vi "Scannig-Probe-Microscope-Controller-2010-03-08-RFR-1a-version-for-MCL-drift-trial-fm-multiple-channels-nanoh50.vi"() -> ()   [LabVIEW 2012]
uses:
  <vilib>/rvi/eio/common/nirviEmuTemplateMethod_errors.vi
  <vilib>/rvi/Emulation/niFpgaSctlEmulationGetInTimedLoop.vi
  <vilib>/rvi/Emulation/niFpgaSctlEmulationGlobalWrite.vi
  <vilib>/rvi/interface/RandomDataEmulation/nirviRandomDataFPGAFIFO.vi
  <vilib>/rvi/interface/RandomDataEmulation/niFpgaRandomDataHandleErrors.vi
  <vilib>/eio/EIONode/EIONode.xnode
  <vilib>/rvi/Analysis/measure/butterworth/XNode/niFpgaButterworthFilter.xnode
  <vilib>/rvi/DataTransferAndStorage/Container/XNode/niFpgaContainer.xnode
  <vilib>/rvi/interface/RandomDataEmulation/nirviRandomDataFpgaReadWriteTemplate.vi
panel:
  in  "Direction":bool
  in  "Enable":bool
  out "Dir":bool
  out "En":bool
  in  "Change Dir / Enable":bool
  in  "Stepper Motor Stop":bool
  in  "Step Motor Cycle (usec)":u32 caption="Stepper Motor Cycle"
  out "Step":bool
  in  "Manual-fixed-steps":i32
  in  "Continuous/Fixed":bool
  in  "Stepper Motor":bool
  in  "Timeout":i32=-1
  in  "acquisition rate calibration":u32 caption="Count(uSec)"
  in  "Manual control Output Calibration":i16
  in  "Wait before\ncalibration":u32 caption="Count(uSec)"
  in  "Size-calibration":i32
  in  "Calibration-period":u32 caption="Count(uSec)"
  in  "Initial Position\n Calibration":i32
  in  "AO1":i16
  in  "Start calibration":bool
  out "AI4":i16
  out "AI2":i16
  out "AI6":i16
  out "AI5":i16
  in  "P scale":i8=-1
  in  "offset retraction drift":i16
  in  "time before averaging drift":u32 caption="Count(uSec)"
  in  "Setpoint Control":bool
  in  "Internal Setpoint Internal Control":i16
  in  "Internal Setpoint External Control":i16=357
  in  "Stop Feedback Control":bool
  in  "shift integrator control":i32
  in  "shift integrator":i32
  out "offset out":i16
  in  "drift temporal control":u32
  in  "offset FM":u16
  in  "drift averager":u16
  out "TF-drift":i16
  out "Counter Data":i8 min=-1 step=1
  in  "drift Waiting (uSec)":u16
  out "End of image":bool
  in  "Pixels in one image":i32
  in  "Scanning Y indicator":bool
  in  "Stop Feedback":bool
  in  "Steps per Feedback Region":i32=665
  in  "Y Number of Lines":u32=10
  in  "PID gains (x 2^8)":T1={"proportional gain (Kc)"=1, "integral gain (Kc*Ts/Ti)"=0, "derivative gain (Kc*Td/Ts)"=0}
  out "Command Out":i16=-4104
  in  "provisional limit":i8=102
  out "accumulator limit":i8=-1
  in  "shift-divisions (always >=2)":i8=100
  out "limit indicator":u8
  in  "counter":i8 min=-1 step=1
  in  "Internal Setpoint":i16=357
  in  "I scale":i8=-1
  in  "Count(uSec)":u8=232
  in  "Timeout FIFO":i32=-1
  out "Y line":i32
  out "iterations x":i32
  out "X Output Value":i16=3
  in  "Forth/Back Y axis":bool
  out "Inidicator \nforth/back  Y axis":i8=1
  in  "Time per step/\nX axis sub pixel (uSec)":u16=31 caption="Count(uSec)"
  in  "Time per image pixel/\nX axis pixel (uSec)":u16=1984 caption="Count(uSec)"
  in  "Time per step/\nY axis sub pixel (uSec)":u32=7936 caption="Count(uSec)"
  out "Y Output Value":i16=32702
  out "End of scan line?":bool
  in  "Forth/Back X axis":bool
  in  "Image Total Pixels":u32=65536
  out "Indicator \nforth/back X axis":i8=1
  in  "Y axis pixels":u16=255
  in  "Y steps per pixel":u16=64
  in  "X steps per pixel":u16=64
  in  "y initial":i16
  in  "x initial":i16
  in  "X axis pixels":u16=255
  in  "Scanning On/Off":bool
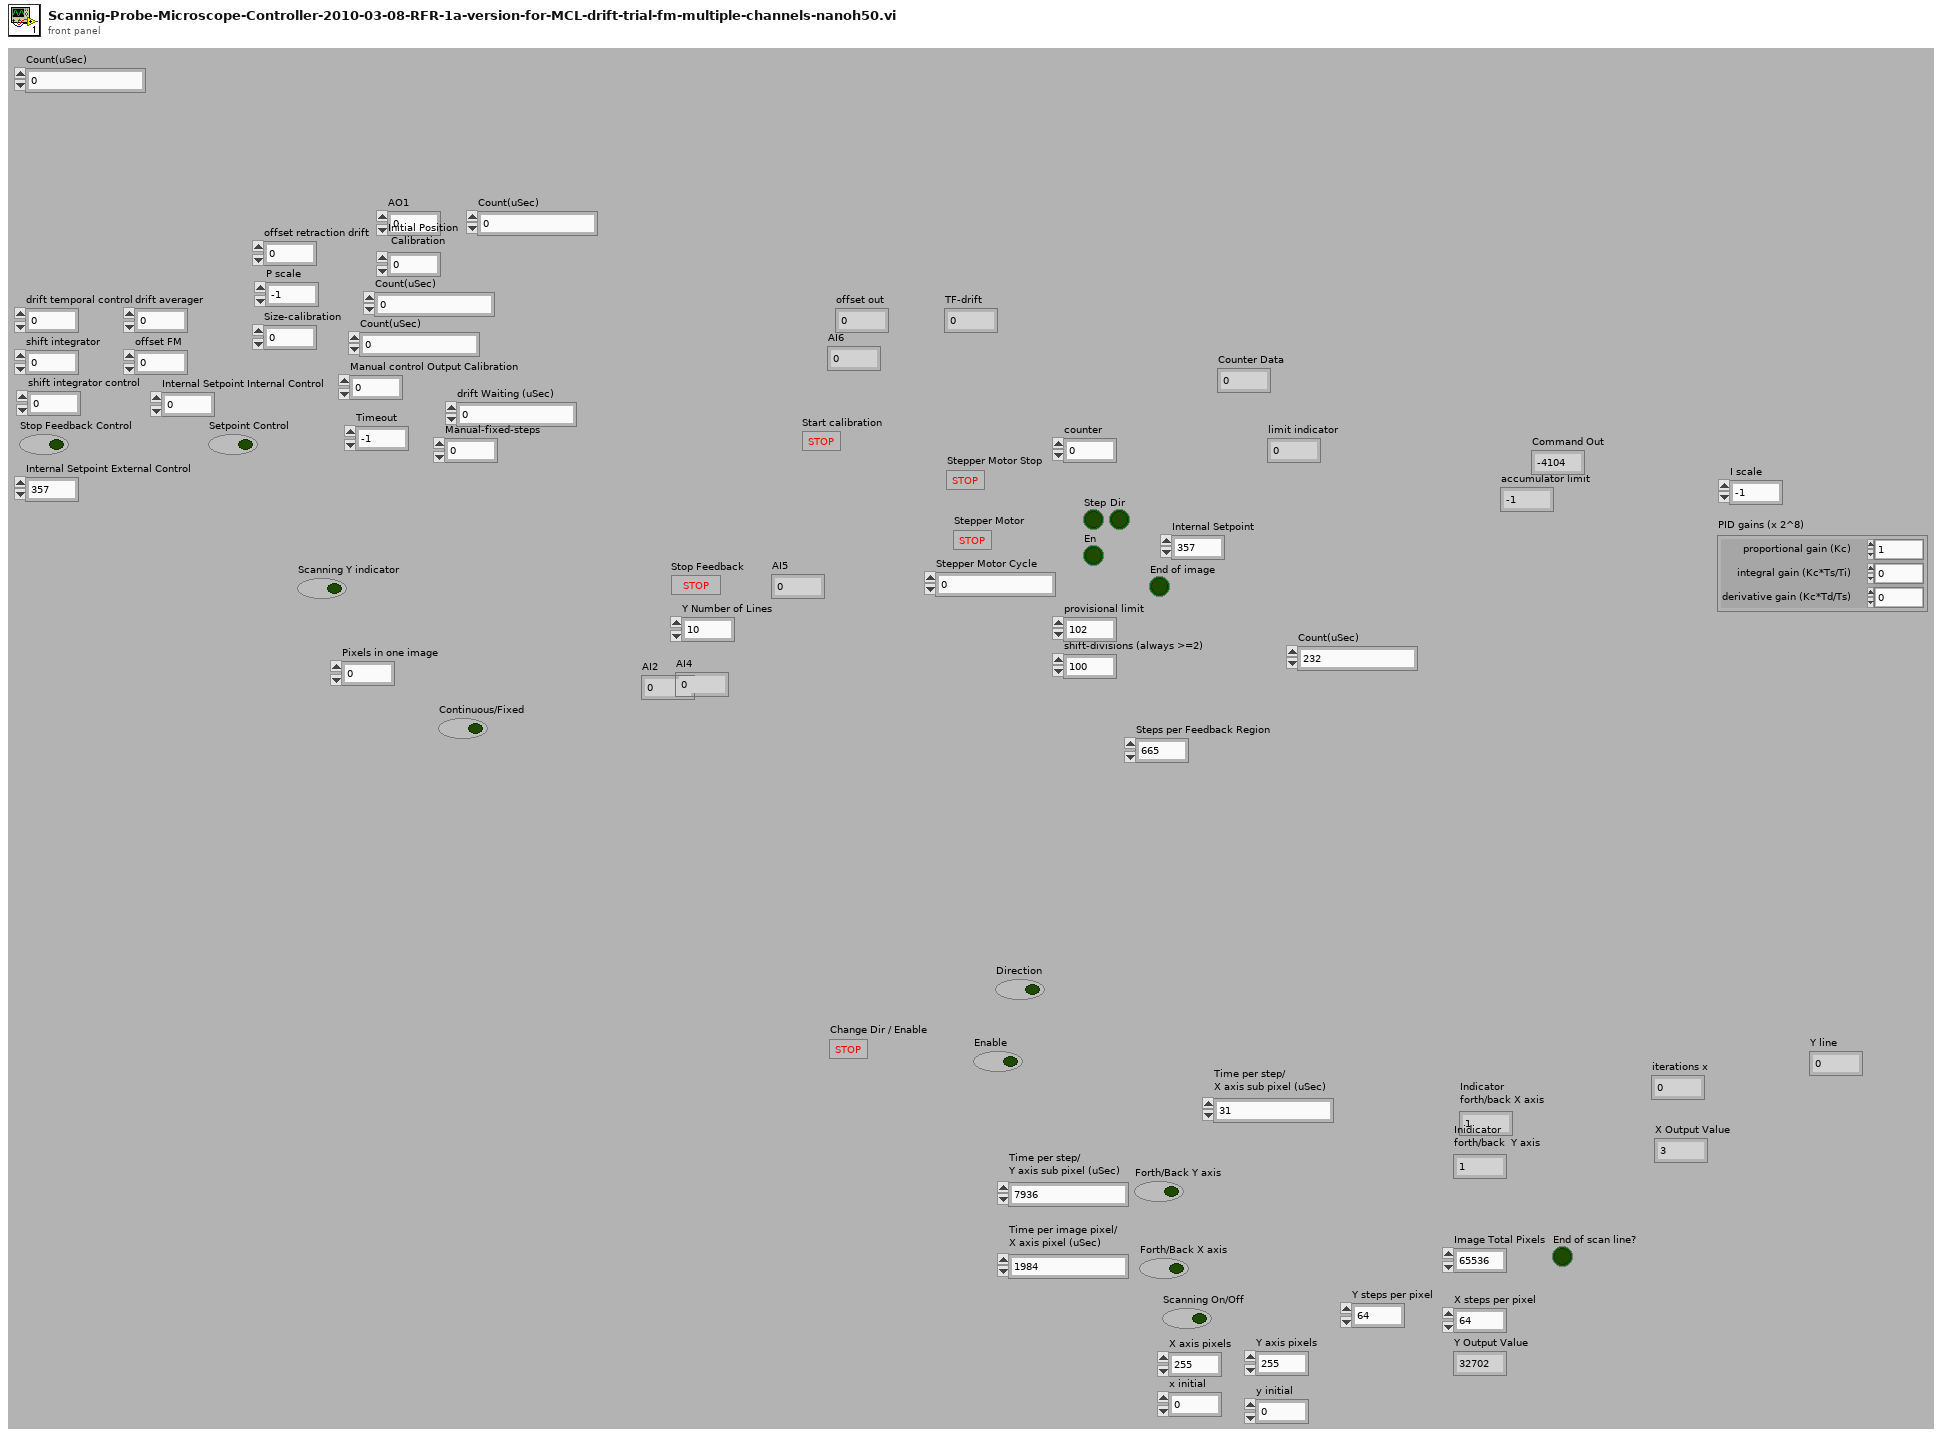
[diagram p1: front panel]
types:
  T1 = cluster{"proportional gain (Kc)":i16, "integral gain (Kc*Ts/Ti)":i16, "derivative gain (Kc*Td/Ts)":i16}
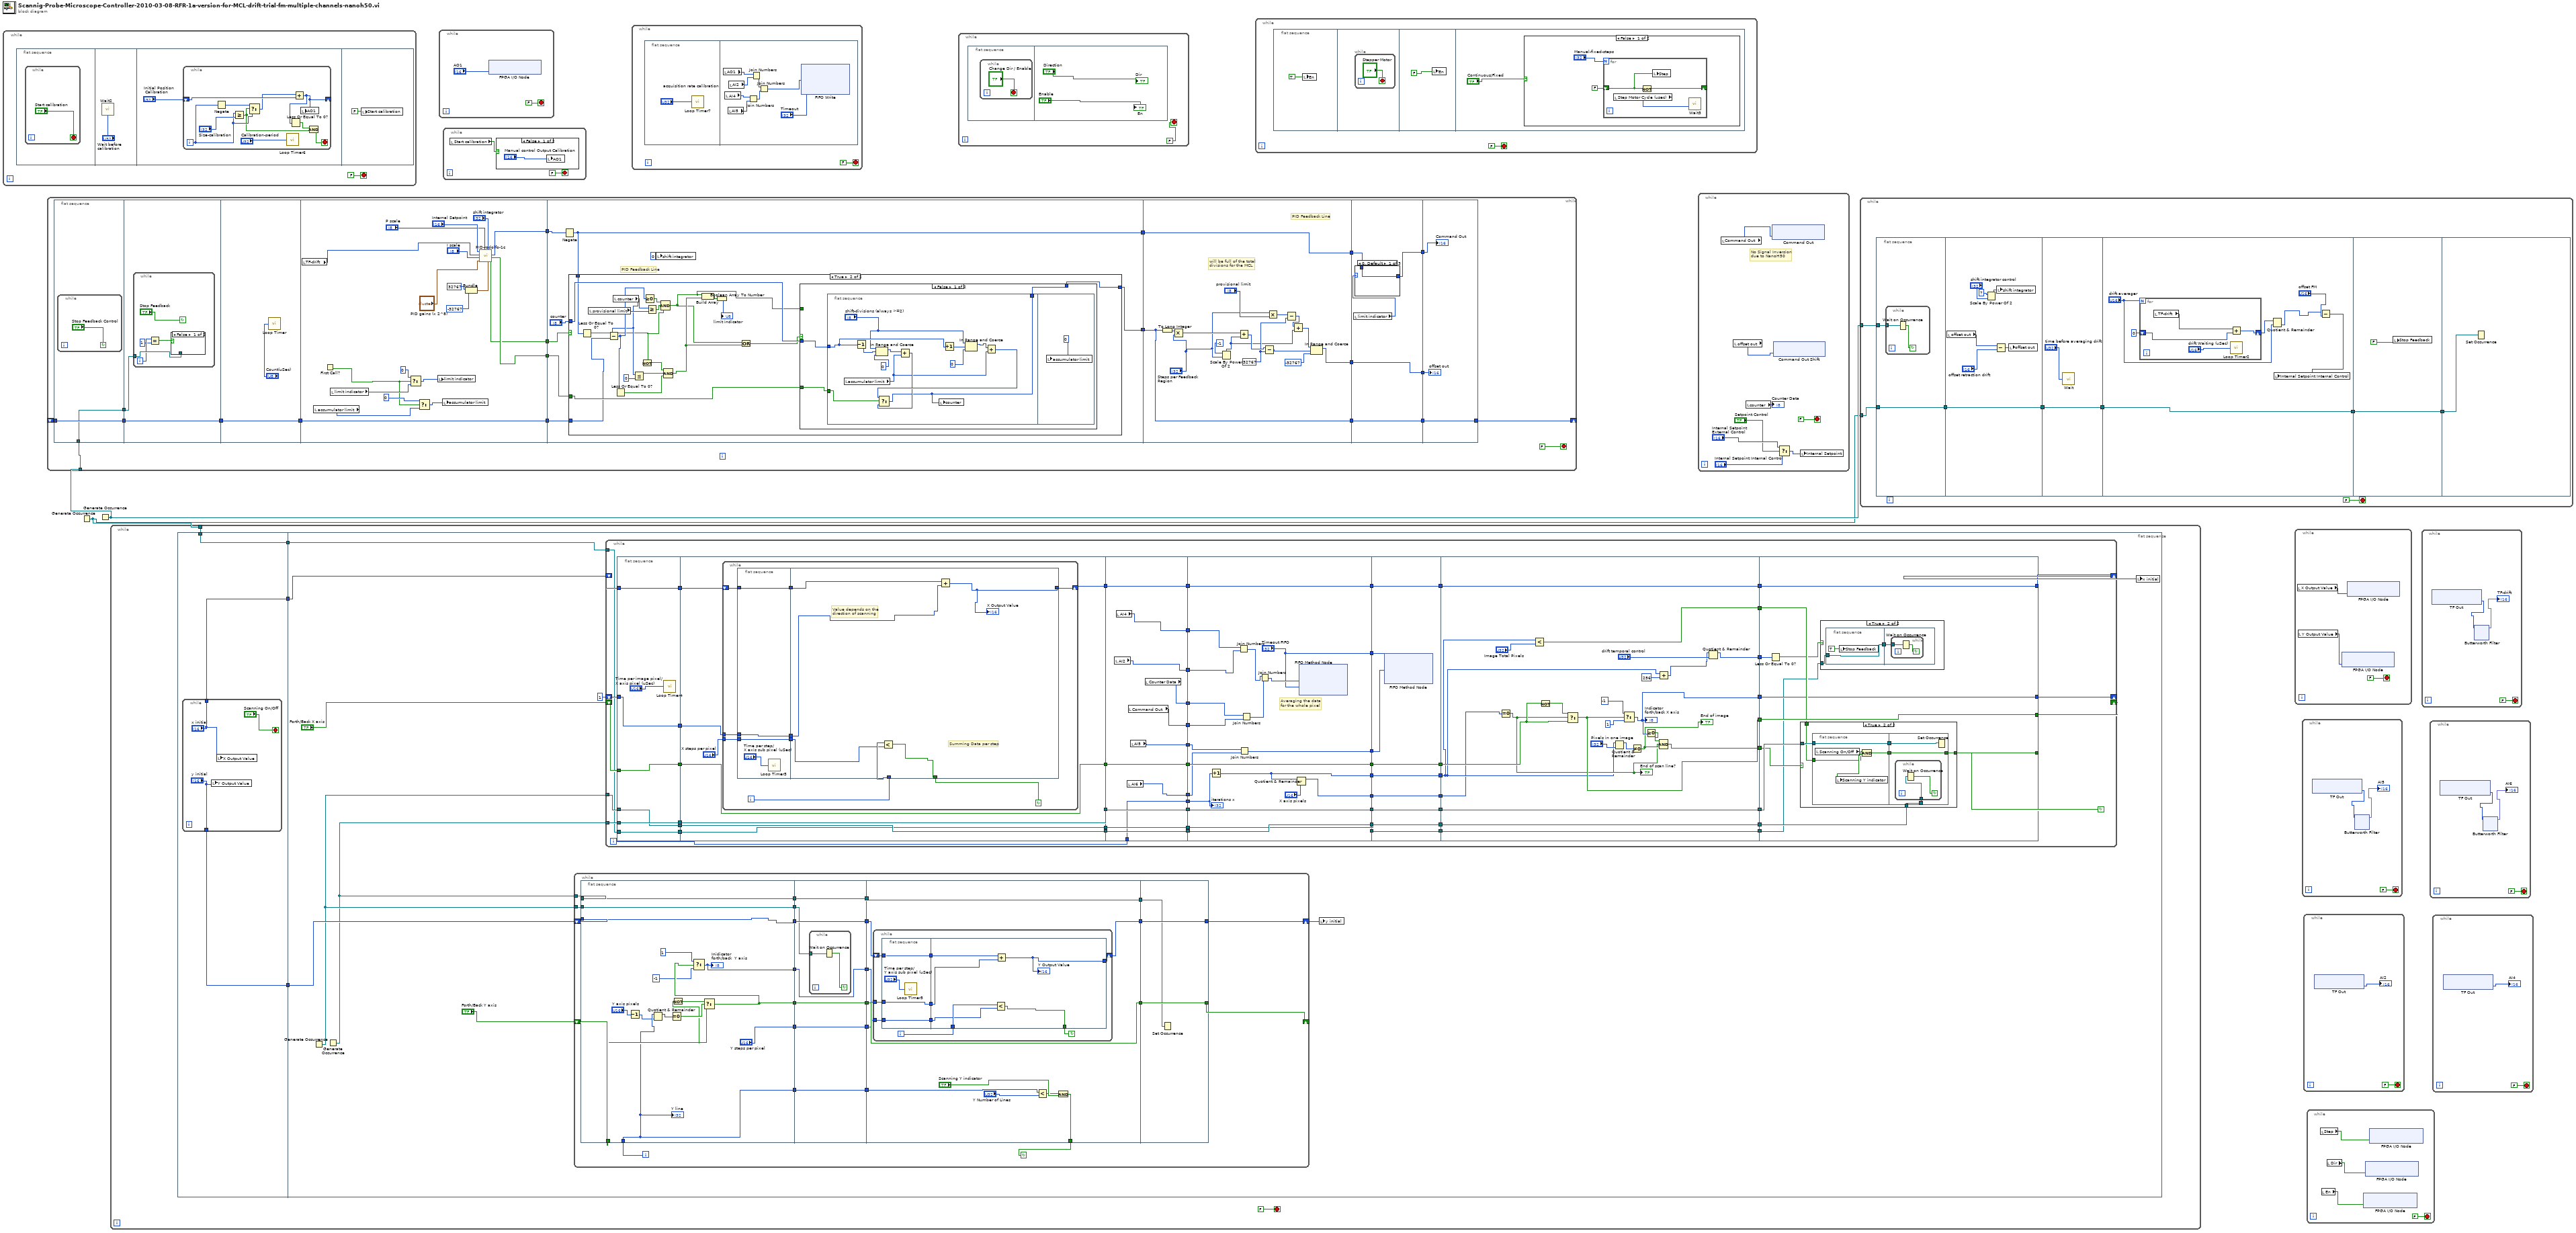
[diagram p0: block diagram]
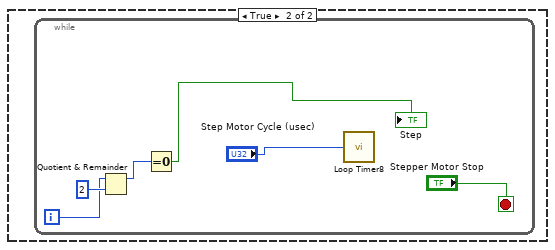
[diagram p2: hidden frame]
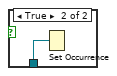
[diagram p4: hidden frame]
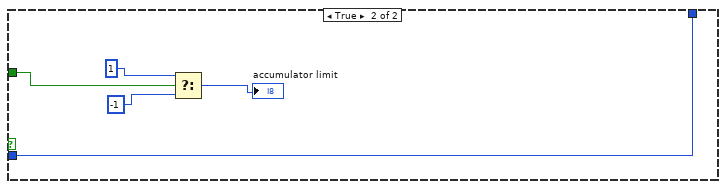
[diagram p6: hidden frame]
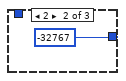
[diagram p7: hidden frame]
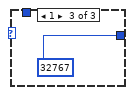
[diagram p8: hidden frame]
diagram:
  n1 = while {
    stop <- FALSE stop-if-true
    n2 = flat-sequence {
      frame #0 {
        n3 = while {
          stop <- "Start calibration" stop-if-true
        }
      }
      frame #1 {
        n4 = call "Wait2"("Count(uSec)"="Wait before\ncalibration") -> ()  [unwired: 1 out]
      }
      frame #2 {
        n5 = while {
          shift-right: [w10] -> _
          shift-left: "Initial Position\n Calibration" -> [w16]
          i -> [w11]
          stop <- w7 stop-if-true
          n6 = Negate(x=w11) -> (-x=w14:i32)
          n7 = Greater Or Equal?(x=w11, y="Size-calibration") -> (x >= y?=w8:bool)
          n8 = Select(t=w14, s=w8, f=w11) -> (s? t:f=w12:i32)
          n9 = call "Loop Timer6"("Count(uSec)"="Calibration-period") -> ()  [unwired: 1 out]
          n10 = Add(x=w12, y=w16) -> (x+y=w10:i32)
          n11 = Less Or Equal To 0?(x=w10) -> (x <= 0?=w9:bool)
          n12 = local write "AO1"(w10) -> ()
          n13 = Compound Arithmetic op=AND(w9, w8) -> (w7:bool)
        }
      }
      frame #3 {
        n14 = local write "Start calibration"(FALSE ("Start calibration")) -> ()
      }
    }
  }
  n15 = Generate Occurrence() -> (w1:refnum<k4>)
  n16 = Generate Occurrence() -> (w2:refnum<k4>)
  n17 = while {
    shift-right: [w28] -> _
    shift-left: _ -> [w27]
    tunnel: w2 -> [w19]
    stop <- FALSE stop-if-true
    n18 = flat-sequence {
      tunnel: w27 -> [w39]
      tunnel: [w39] -> w21
      tunnel: w19 -> [w38]
      tunnel: [w38] -> w18
      tunnel: w21 -> [w42]
      tunnel: [w42] -> w20
      tunnel: w18 -> [w41]
      tunnel: [w49] -> w26
      tunnel: w20 -> [w49]
      tunnel: [w67] -> w25
      tunnel: [w66] -> w24
      tunnel: [w65] -> w23
      tunnel: w26 -> [w62]
      tunnel: [w62] -> w22
      tunnel: [w78] -> w31
      tunnel: w25 -> [w77]
      tunnel: [w73] -> w32
      tunnel: w24 -> [w75]
      tunnel: w23 -> [w74]
      tunnel: w22 -> [w72]
      tunnel: w32 -> [w135]
      tunnel: [w135] -> w34
      tunnel: w31 -> [w132]
      tunnel: [w133] -> w33
      tunnel: [w132] -> w30
      tunnel: [w139] -> w36
      tunnel: w34 -> [w141]
      tunnel: [w142] -> w35
      tunnel: w33 -> [w139]
      tunnel: w30 -> [w138]
      tunnel: [w138] -> w29
      tunnel: w36 -> [w146]
      tunnel: w35 -> [w148]
      tunnel: w29 -> [w147]
      tunnel: [w147] -> w28
      frame #0 {
        n19 = while {
          stop <- "Stop Feedback Control" continue-if-true
        }
      }
      frame #1 {
        n20 = while {
          tunnel: w41 -> [w47]
          i -> [w45]
          stop <- "Stop Feedback" continue-if-true
          n21 = Equal?(x=w45, y=u8 1) -> (x = y?=w43:bool)
          n22 = case shown="False" w43 {
            tunnel: w47 -> [_ w48]
            frame False {
            }
            frame True {
              n23 = Set Occurrence(w48) -> ()
            }
          }
        }
      }
      frame #2 {
        n24 = call "Loop Timer"("Count(uSec)"="Count(uSec)") -> ()  [unwired: 1 out]
      }
      frame #3 {
        n25 = local read "TF-drift"() -> (w52:i16)
        n26 = local read "accumulator limit"() -> (w55:i8)
        n27 = First Call?() -> (First Call?: T/F=w53:bool)
        n28 = local read "limit indicator"() -> (w58:u8)
        n29 = Select(t=u8 0, s=w53, f=w58) -> (s? t:f=w59:u8)
        n30 = Select(t=i8 0, s=w53, f=w55) -> (s? t:f=w57:i8)
        n31 = local write "limit indicator"(w59) -> ()
        n32 = local write "accumulator limit"(w57) -> ()
        n33 = Bundle(i16 32767, i16 -32767) -> (w68:cluster{i16, i16})  [unwired: 1 in]
        n34 = call "PID-rodolfo-1c.vi"("output range"=w68, "shift integrator"="shift integrator", "P scale"="P scale", "PID gains (x 2^8)"="PID gains (x 2^8)", "I scale"="I scale", "process variable"=w52, "setpoint"="Internal Setpoint") -> ("yes/no"=w65:bool, "upper/lower"=w66:bool, "output"=w67:i16)  [unwired: 2 in]
      }
      frame #4 {
        # "PID Feedback Line"
        n35 = Negate(x=w77) -> (-x=w73:i16)
        n36 = case shown="True" w74 {
          tunnel: "counter" -> [w79 w99]
          tunnel: [w79 w98] -> w78
          tunnel: w75 -> [_ w82]
          tunnel: w73 -> [_ w87]
          tunnel: w72 -> [_ w80]
          frame False {
          }
          frame True {
            n37 = Less Or Equal To 0?(x=w87) -> (x <= 0?=w88:bool)
            n38 = local read "provisional limit"() -> (w95:i8)
            n39 = local read "counter"() -> (w90:i8)
            n40 = Subtract(x=w90, y=w80) -> (x-y=w91:i8)
            n41 = Less Or Equal To 0?(x=w91) -> (x <= 0?=w92:bool)
            n42 = Less Or Equal?(x=w90, y=u8 0) -> (x <= y?=w93:bool)
            n43 = Not(x=w88) -> (.not. x?=w89:bool)
            n44 = Greater Or Equal To 0?(x=w91) -> (x >= 0?=w97:bool)
            n45 = Greater Or Equal?(x=w90, y=w95) -> (x >= y?=w96:bool)
            n46 = Compound Arithmetic op=AND(w97, w96, w88) -> (w81:bool)
            n47 = Compound Arithmetic op=AND(w89, w93, w92) -> (w84:bool)
            n48 = Build Array(w81, w84) -> (w86:bool[])
            n49 = Boolean Array To Number(Boolean array=w86) -> (number=→"limit indicator":u8)
            n50 = Or(x=w81, y=w84) -> (x .or. y?=w83:bool)
            n51 = case shown="False" w83 {
              tunnel: w99 -> [w102 w121]
              tunnel: [w101 w121] -> w98
              tunnel: w82 -> [w100 _]
              tunnel: w81 -> [_ w117]
              frame False {
                n52 = flat-sequence {
                  tunnel: w102 -> [w108]
                  tunnel: [w105] -> w101
                  tunnel: w100 -> [w109]
                  frame #0 {
                    n53 = local read "accumulator limit"() -> (w104:i8)
                    n54 = Decrement(x=w108) -> (x-1=w112:i8)
                    n55 = In Range and Coerce(upper limit="shift-divisions (always >=2)", x=w112, lower limit=i8 0) -> (coerced(x)=w110:i8)  [unwired: 1 out]
                    n56 = Add(x=w110, y=w104) -> (x+y=w106:i8)
                    n57 = Increment(x=w108) -> (x+1=w113:i8)
                    n58 = In Range and Coerce(upper limit="shift-divisions (always >=2)", x=w113, lower limit=i8 0 ("y")) -> (coerced(x)=w115:i8)  [unwired: 1 out]
                    n59 = Add(x=w115, y=w104) -> (x+y=w107:i8)
                    n60 = Select(t=w107, s=w109, f=w106) -> (s? t:f=w105:i8)
                    n61 = local write "counter"(w105) -> ()
                  }
                  frame #1 {
                    n62 = local write "accumulator limit"(i8 0 ("accumulator limit")) -> ()
                  }
                }
              }
              frame True {
                n63 = Select(t=i8 1, s=w117, f=i8 -1) -> (s? t:f=→"accumulator limit":i8)
              }
            }
          }
        }
        n64 = local write "shift integrator"(0 ("new integrator")) -> ()
      }
      frame #5 {
        w125 = 32767 ("y")
        # "PID Feedback Line"
        # "will be full of the total\ndivisions for the MCL"
        n65 = To Long Integer(number=w132) -> (32bit integer=w131:i32)
        n66 = Multiply(x=w131, y="Steps per Feedback Region") -> (x*y=w136:i32)
        n67 = Scale By Power Of 2(n=i8 -1, x="Steps per Feedback Region") -> (x*2^n=w124:i32)
        n68 = Add(x=w136, y=w124) -> (x+y=w128:i32)
        n69 = Subtract(x=w128, y=w125) -> (x-y=w127:i32)
        n70 = Multiply(x="Steps per Feedback Region", y="provisional limit") -> (x*y=w126:i32)
        n71 = Subtract(x=w126, y=w125) -> (x-y=w123:i32)
        n72 = Add(x=w123, y=w124) -> (x+y=w122:i32)
        n73 = In Range and Coerce(upper limit=w122, x=w127, lower limit=-32767) -> (coerced(x)=w133:i32)  [unwired: 1 out]
      }
      frame #6 {
        n74 = local read "limit indicator"() -> (w140:u8)
        n75 = case shown="0, Default" w140 {
          tunnel: w141 -> [w143 _ _]
          tunnel: [w143 i16 -32767 i16 32767] -> w142
          frame 0, Default {
          }
          frame 2 {
          }
          frame 1 {
          }
        }
      }
      frame #7 {
        "Command Out" <- w148
        "offset out" <- w146
      }
    }
  }
  n76 = while {
    tunnel: w1 -> [w149]
    stop <- FALSE stop-if-true
    n77 = flat-sequence {
      tunnel: [w155] -> w152
      tunnel: [w156] -> w151
      tunnel: [w154] -> w150
      tunnel: w149 -> [w154]
      tunnel: w152 -> [w165]
      tunnel: w151 -> [w164]
      tunnel: w150 -> [w160]
      frame #0 {
        n78 = while {
          tunnel: ["y initial"] -> w156
          tunnel: ["x initial"] -> w155
          stop <- "Scanning On/Off" stop-if-true
          n79 = local write "Y Output Value"("y initial") -> ()
          n80 = local write "X Output Value"("x initial") -> ()
        }
      }
      frame #1 {
        n81 = Generate Occurrence() -> (w163:refnum<k4>)
        n82 = Generate Occurrence() -> (w162:refnum<k4>)
        n83 = while {
          shift-right: [w193] -> _
          shift-left: "Forth/Back Y axis" -> [w192]
          shift-right: [w190] -> w166
          shift-left: w164 -> [w191]
          tunnel: w163 -> [w189]
          tunnel: w162 -> [w185]
          i -> [w173]
          stop <- w172 continue-if-true
          n84 = flat-sequence {
            tunnel: w192 -> [w206]
            tunnel: [w204] -> w184
            tunnel: [w201] -> w182
            tunnel: [w200] -> w180
            tunnel: [w199] -> w178
            tunnel: ["Y steps per pixel"] -> w176
            tunnel: [w197] -> w174
            tunnel: w173 -> [w196]
            tunnel: w191 -> [w201]
            tunnel: w185 -> [w199]
            tunnel: w189 -> [w197]
            tunnel: [w196] -> w170
            tunnel: w184 -> [w215]
            tunnel: [w215] -> w183
            tunnel: w182 -> [w214]
            tunnel: [w214] -> w181
            tunnel: w180 -> [w213]
            tunnel: [w213] -> w179
            tunnel: w178 -> [w212]
            tunnel: [w212] -> w177
            tunnel: w176 -> [w211]
            tunnel: [w211] -> w175
            tunnel: w174 -> [w210]
            tunnel: [w209] -> w171
            tunnel: w170 -> [w209]
            tunnel: w183 -> [w228]
            tunnel: w181 -> [w227]
            tunnel: w179 -> [w225]
            tunnel: [w228] -> w188
            tunnel: [w226] -> w187
            tunnel: [w224] -> w186
            tunnel: w177 -> [w224]
            tunnel: w175 -> [w223]
            tunnel: [w219] -> w172
            tunnel: w171 -> [w218]
            tunnel: [w249] -> w190
            tunnel: [w250] -> w193
            tunnel: w188 -> [w250]
            tunnel: w187 -> [w249]
            tunnel: w186 -> [w248]
            frame #0 {
              n85 = Decrement(x="Y axis pixels") -> (x-1=w194:u16)
              n86 = Quotient & Remainder(x=w196, y=w194) -> (x-y*floor(x/y)=w208:i32)  [unwired: 1 out]
              n87 = Equal To 0?(x=w208) -> (x = 0?=w207:bool)
              n88 = Not(x=w206) -> (.not. x?=w205:bool)
              n89 = Select(t=w205, s=w207, f=w206) -> (s? t:f=w204:bool)
              n90 = Select(t=i8 1, s=w204, f=i8 -1 ("Inidicator \nforth/back  Y axis")) -> (s? t:f=w200:i8)
              "Inidicator \nforth/back  Y axis" <- w200
              "Y line" <- w196
            }
            frame #1 {
              n91 = while {
                tunnel: w210 -> [w216]
                stop <- w217 continue-if-true
                n92 = Wait on Occurrence(2:w216) -> (0:w217:bool)  [unwired: 2 in]
              }
            }
            frame #2 {
              n93 = while {
                shift-right: [w234] -> w226
                shift-left: w227 -> [w235]
                tunnel: w225 -> [w231]
                tunnel: w223 -> [w229]
                i -> [w236]
                stop <- w237 continue-if-true
                n94 = flat-sequence {
                  tunnel: w235 -> [w241]
                  tunnel: [w241] -> w233
                  tunnel: [w239] -> w232
                  tunnel: w231 -> [w239]
                  tunnel: [w238] -> w230
                  tunnel: w229 -> [w238]
                  tunnel: [w243] -> w237
                  tunnel: w236 -> [w247]
                  tunnel: [w245] -> w234
                  tunnel: w233 -> [w246]
                  tunnel: w232 -> [w244]
                  tunnel: w230 -> [w242]
                  frame #0 {
                    n95 = call "Loop Timer5"("Count(uSec)"="Time per step/\nY axis sub pixel (uSec)") -> ()  [unwired: 1 out]
                  }
                  frame #1 {
                    n96 = Less?(x=w247, y=w242) -> (x < y?=w243:bool)
                    n97 = Add(x=w246, y=w244) -> (x+y=w245:i16)
                    "Y Output Value" <- w245
                  }
                }
              }
              n98 = Less?(x=w218, y="Y Number of Lines") -> (x < y?=w220:bool)
              n99 = Compound Arithmetic op=AND(w220, "Scanning Y indicator") -> (w219:bool)
            }
            frame #3 {
              n100 = Set Occurrence(w248) -> ()
            }
          }
        }
        n101 = while {
          shift-right: [w307] -> w167
          shift-left: w165 -> [w309]
          shift-right: [w294] -> _
          shift-left: "Forth/Back X axis" -> [w308]
          tunnel: w163 -> [w306]
          tunnel: w162 -> [w305]
          shift-right: [w296] -> _
          shift-left: i8 1 ("Indicator \nforth/back") -> [w295]
          tunnel: w160 -> [w275]
          i -> [w267]
          stop <- w304 continue-if-true
          n102 = flat-sequence {
            tunnel: w308 -> [w315]
            tunnel: w309 -> [w316]
            tunnel: [w316] -> w293
            tunnel: [w315] -> w292
            tunnel: w306 -> [w313]
            tunnel: [w313] -> w291
            tunnel: [w312] -> w290
            tunnel: w305 -> [w312]
            tunnel: [w311] -> w289
            tunnel: w295 -> [w311]
            tunnel: w275 -> [w310]
            tunnel: [w310] -> w271
            tunnel: w293 -> [w322]
            tunnel: [w324] -> w288
            tunnel: [w321] -> w282
            tunnel: w290 -> [w321]
            tunnel: [w320] -> w280
            tunnel: w291 -> [w320]
            tunnel: [w319] -> w278
            tunnel: w292 -> [w319]
            tunnel: w289 -> [w323]
            tunnel: [w317] -> w272
            tunnel: w271 -> [w317]
            tunnel: w288 -> [w355]
            tunnel: [w355] -> w287
            tunnel: [w344] -> w286
            tunnel: [w345] -> w285
            tunnel: [w350] -> w284
            tunnel: [w351] -> w283
            tunnel: w282 -> [w354]
            tunnel: [w354] -> w281
            tunnel: w280 -> [w353]
            tunnel: [w353] -> w279
            tunnel: w278 -> [w352]
            tunnel: [w352] -> w277
            tunnel: [w349] -> w273
            tunnel: w272 -> [w349]
            tunnel: [w346] -> w270
            tunnel: [w347] -> w269
            tunnel: [w348] -> w268
            tunnel: w267 -> [w348]
            tunnel: w287 -> [w375]
            tunnel: w286 -> [w367]
            tunnel: w285 -> [w366]
            tunnel: w284 -> [w371]
            tunnel: w283 -> [w365]
            tunnel: [w375] -> w266
            tunnel: [w370] -> w264
            tunnel: w281 -> [w370]
            tunnel: [w369] -> w262
            tunnel: w279 -> [w369]
            tunnel: [w368] -> w260
            tunnel: w277 -> [w368]
            tunnel: [w364] -> w258
            tunnel: w273 -> [w364]
            tunnel: w270 -> [w363]
            tunnel: w269 -> [w362]
            tunnel: w268 -> [w361]
            tunnel: [w359] -> w256
            tunnel: [w358] -> w254
            tunnel: ["Timeout FIFO"] -> w252
            tunnel: [w356] -> w251
            tunnel: w266 -> [w384]
            tunnel: [w384] -> w265
            tunnel: w264 -> [w383]
            tunnel: [w383] -> w263
            tunnel: w262 -> [w382]
            tunnel: [w382] -> w261
            tunnel: w260 -> [w381]
            tunnel: [w381] -> w259
            tunnel: w258 -> [w380]
            tunnel: [w380] -> w257
            tunnel: w256 -> [w379]
            tunnel: [w379] -> w255
            tunnel: w254 -> [w378]
            tunnel: [w378] -> w253
            tunnel: w252 -> [w377]
            tunnel: w251 -> [w376]
            tunnel: [w400] -> w303
            tunnel: w265 -> [w408]
            tunnel: [w408] -> w302
            tunnel: w263 -> [w407]
            tunnel: [w407] -> w301
            tunnel: w261 -> [w406]
            tunnel: [w406] -> w300
            tunnel: [w401] -> w299
            tunnel: w259 -> [w399]
            tunnel: [w398] -> w298
            tunnel: [w397] -> w297
            tunnel: [w390] -> w276
            tunnel: [w387] -> w274
            tunnel: w257 -> [w387]
            tunnel: w255 -> [w386]
            tunnel: w253 -> [w385]
            tunnel: [w418] -> w307
            tunnel: [w419] -> w294
            tunnel: w303 -> [w419]
            tunnel: w302 -> [w418]
            tunnel: w301 -> [w417]
            tunnel: w300 -> [w416]
            tunnel: w299 -> [w415]
            tunnel: [w414] -> w304
            tunnel: w298 -> [w413]
            tunnel: [w412] -> w296
            tunnel: w297 -> [w412]
            tunnel: w276 -> [w411]
            tunnel: w274 -> [w409]
            frame #0 {
              n103 = call "Loop Timer4"("Count(uSec)"="Time per image pixel/\nX axis pixel (uSec)") -> ()  [unwired: 1 out]
            }
            frame #1 {
              n104 = while {
                shift-right: [w330] -> w324
                shift-left: w322 -> [w331]
                tunnel: w323 -> [w327]
                tunnel: "X steps per pixel" -> [w325]
                i -> [w332]
                stop <- w333 continue-if-true
                n105 = flat-sequence {
                  tunnel: w331 -> [w337]
                  tunnel: [w337] -> w329
                  tunnel: [w335] -> w328
                  tunnel: w327 -> [w335]
                  tunnel: [w334] -> w326
                  tunnel: w325 -> [w334]
                  tunnel: [w339] -> w333
                  tunnel: w332 -> [w343]
                  tunnel: [w341] -> w330
                  tunnel: w329 -> [w342]
                  tunnel: w328 -> [w340]
                  tunnel: w326 -> [w338]
                  frame #0 {
                    n106 = call "Loop Timer3"("Count(uSec)"="Time per step/\nX axis sub pixel (uSec)") -> ()  [unwired: 1 out]
                  }
                  frame #1 {
                    # "Summing Data per step"
                    # "Value depends on the\ndirection of scanning"
                    n107 = Less?(x=w343, y=w338) -> (x < y?=w339:bool)
                    n108 = Add(x=w342, y=w340) -> (x+y=w341:i16)
                    "X Output Value" <- w341
                  }
                }
              }
            }
            frame #2 {
              n109 = local read "AI2"() -> (w345:i16)
              n110 = local read "AI4"() -> (w344:i16)
              n111 = local read "AI6"() -> (w347:i16)
              n112 = local read "Command Out"() -> (w351:i16)
              n113 = local read "AI5"() -> (w346:i16)
              n114 = local read "Counter Data"() -> (w350:i8)
            }
            frame #3 {
              # "Averaging the data \nfor the whole pixel"
              n115 = Increment(x=w361) -> (x+1=w359:i32)
              n116 = Join Numbers(hi=w367, lo=w366) -> ((hi.lo)=w372:u32)
              n117 = Join Numbers(hi=w363, lo=w362) -> ((hi.lo)=w356:u32)
              n118 = Join Numbers(hi=w371, lo=w365) -> ((hi.lo)=w373:u32)
              n119 = Join Numbers(hi=w372, lo=w373) -> ((hi.lo)=w374:u64)
              n120 = Quotient & Remainder(x=w359, y="X axis pixels") -> (x-y*floor(x/y)=w358:i32)  [unwired: 1 out]
              n121 = xnode "FIFO Method Node"("Element"=w374, "Timeout"="Timeout FIFO") -> ()  [unwired: 1 in, 2 out]
              "iterations x" <- w361
            }
            frame #4 {
              n122 = xnode ("FIFO Method Node")("Element"=w376, "Timeout"=w377) -> ()  [unwired: 1 in, 2 out]
            }
            frame #5 {
              n123 = Equal To 0?(x=w385) -> (x = 0?=w393:bool)
              "End of scan line?" <- w393
              n124 = Less?(x=w386, y="Image Total Pixels") -> (x < y?=w401:bool)
              n125 = Not(x=w399) -> (.not. x?=w405:bool)
              n126 = Select(t=w405, s=w393, f=w399) -> (s? t:f=w400:bool)
              n127 = Quotient & Remainder(x=w386, y="Pixels in one image") -> (x-y*floor(x/y)=w394:i32)  [unwired: 1 out]
              n128 = Select(t=i8 -1 ("Indicator \nforth/back"), s=w400, f=i8 1 ("Indicator \nforth/back")) -> (s? t:f=w397:i8)
              "Indicator \nforth/back X axis" <- w397
              n129 = Not Equal To 0?(x=w394) -> (x != 0?=w396:bool)
              "End of image" <- w396
              n130 = Greater Or Equal To 0?(x=w397) -> (x >= 0?=w392:bool)
              n131 = Add(x=w386, y=u16 256) -> (x+y=w388:i32)
              n132 = Compound Arithmetic op=AND(w392, w393, w396) -> (w398:bool)
              n133 = Quotient & Remainder(x=w388, y="drift temporal control") -> (x-y*floor(x/y)=w390:u32)  [unwired: 1 out]
            }
            frame #6 {
              n134 = Less Or Equal To 0?(x=w411) -> (x <= 0?=w410:bool)
              n135 = case shown="True" w413 {
                tunnel: w416 -> [_ w433]
                tunnel: w417 -> [_ w432]
                tunnel: w415 -> [w427 w430]
                tunnel: [w427 w429] -> w414
                frame False {
                }
                frame True {
                  n136 = flat-sequence {
                    tunnel: w433 -> [w437]
                    tunnel: [w437] -> w431
                    tunnel: w430 -> [w435]
                    tunnel: [w434] -> w428
                    tunnel: w432 -> [w439]
                    tunnel: w431 -> [w440]
                    tunnel: [w438] -> w429
                    tunnel: w428 -> [w438]
                    frame #0 {
                      n137 = local read "Scanning On/Off"() -> (w436:bool)
                      n138 = local write "Scanning Y indicator"(w436) -> ()
                      n139 = Compound Arithmetic op=AND(w435, w436) -> (w434:bool)
                    }
                    frame #1 {
                      n140 = while {
                        tunnel: w439 -> [w441]
                        stop <- w442 continue-if-true
                        n141 = Wait on Occurrence(2:w441) -> (0:w442:bool)  [unwired: 2 in]
                      }
                      n142 = Set Occurrence(w440) -> ()
                    }
                  }
                }
              }
              n143 = case shown="True" w410 {
                tunnel: w409 -> [_ w421]
                frame False {
                }
                frame True {
                  n144 = flat-sequence {
                    tunnel: w421 -> [w422]
                    tunnel: [w422] -> w420
                    tunnel: w420 -> [w424]
                    frame #0 {
                      n145 = local write "Stop Feedback"(TRUE ("Stop Feedback")) -> ()
                    }
                    frame #1 {
                      n146 = while {
                        tunnel: w424 -> [w425]
                        stop <- w426 continue-if-true
                        n147 = Wait on Occurrence(2:w425) -> (0:w426:bool)  [unwired: 2 in]
                      }
                    }
                  }
                }
              }
            }
          }
        }
        n148 = local write "y initial"(w166) -> ()
        n149 = local write "x initial"(w167) -> ()
      }
    }
  }
  n150 = while {
    stop <- FALSE stop-if-true
    n151 = xnode "FPGA I/O Node"("Connector0/AO1"="AO1") -> ()  [unwired: 1 in, 1 out]
  }
  n152 = while {
    stop <- FALSE stop-if-true
    n153 = local read "Start calibration"() -> (w446:bool)
    n154 = case shown="False" w446 {
      frame False {
        n155 = local write "AO1"("Manual control Output Calibration") -> ()
      }
      frame True {
      }
    }
  }
  n156 = while {
    stop <- FALSE stop-if-true
    n157 = flat-sequence {
      frame #0 {
        n158 = call "Loop Timer7"("Count(uSec)"="acquisition rate calibration") -> ()  [unwired: 1 out]
      }
      frame #1 {
        n159 = local read "AO1"() -> (w457:i16)
        n160 = local read "AI4"() -> (w454:i16)
        n161 = local read "AI5"() -> (w455:i16)
        n162 = local read "AI2"() -> (w456:i16)
        n163 = Join Numbers(hi=w454, lo=w455) -> ((hi.lo)=w452:u32)
        n164 = Join Numbers(hi=w457, lo=w456) -> ((hi.lo)=w453:u32)
        n165 = Join Numbers(hi=w453, lo=w452) -> ((hi.lo)=w451:u64)
        n166 = xnode ("FIFO Write")("Element"=w451, "Timeout"="Timeout") -> ()  [unwired: 1 in, 2 out]
      }
    }
  }
  n167 = while {
    stop <- FALSE stop-if-true
    n168 = flat-sequence {
      frame #0 {
        n169 = while {
          stop <- "Change Dir / Enable" stop-if-true
        }
      }
      frame #1 {
        "Dir" <- "Direction"
        "En" <- "Enable"
      }
    }
  }
  n170 = while {
    stop <- FALSE stop-if-true
    n171 = flat-sequence {
      frame #0 {
        n172 = local write "En"(TRUE ("Enable")) -> ()
      }
      frame #1 {
        n173 = while {
          stop <- "Stepper Motor" stop-if-true
        }
      }
      frame #2 {
        n174 = local write "En"(FALSE ("Enable")) -> ()
      }
      frame #3 {
        n175 = case shown="False" "Continuous/Fixed" {
          frame False {
            n176 = for {
              N: "Manual-fixed-steps" -> [_]
              shift-right: [w471] -> _
              shift-left: FALSE -> [w469]
              n177 = local read "Step Motor Cycle (usec)"() -> (w470:u32)
              n178 = Not(x=w469) -> (.not. x?=w471:bool)
              n179 = local write "Step"(w469) -> ()
              n180 = call "Wait3"("Count(uSec)"=w470) -> ()  [unwired: 1 out]
            }
          }
          frame True {
            n181 = while {
              i -> [w476]
              stop <- "Stepper Motor Stop" stop-if-true
              n182 = Quotient & Remainder(x=w476, y=u8 2) -> (x-y*floor(x/y)=w475:i32)  [unwired: 1 out]
              n183 = Equal To 0?(x=w475) -> (x = 0?=→"Step":bool)
              n184 = call "Loop Timer8"("Count(uSec)"="Step Motor Cycle (usec)") -> ()  [unwired: 1 out]
            }
          }
        }
      }
    }
  }
  n185 = while {
    stop <- FALSE stop-if-true
    # "No Signal Inversion\ndue to NanoH50"
    n186 = local read "Command Out"() -> (w478:i16)
    n187 = local read "offset out"() -> (w479:i16)
    n188 = local read "counter"() -> (→"Counter Data":i8)
    n189 = xnode "Command Out"("Connector0/AO7"=w478) -> ()  [unwired: 1 in, 1 out]
    n190 = xnode "Command Out Shift"("Connector0/AO2"=w479) -> ()  [unwired: 1 in, 1 out]
    n191 = Select(t="Internal Setpoint External Control", s="Setpoint Control", f="Internal Setpoint Internal Control") -> (s? t:f=w482:i16)
    n192 = local write "Internal Setpoint"(w482) -> ()
  }
  n193 = while {
    tunnel: w2 -> [w493]
    tunnel: w1 -> [w488]
    stop <- FALSE stop-if-true
    n194 = flat-sequence {
      tunnel: w493 -> [w495]
      tunnel: [w494] -> w489
      tunnel: w488 -> [w494]
      tunnel: [w499] -> w487
      tunnel: w489 -> [w499]
      tunnel: w487 -> [w506]
      tunnel: [w506] -> w486
      tunnel: [w512] -> w490
      tunnel: w486 -> [w512]
      tunnel: [w518] -> w491
      tunnel: w490 -> [w518]
      tunnel: w491 -> [w520]
      frame #0 {
        n195 = while {
          tunnel: w495 -> [w496]
          stop <- w497 continue-if-true
          n196 = Wait on Occurrence(2:w496) -> (0:w497:bool)  [unwired: 2 in]
        }
      }
      frame #1 {
        n197 = local read "offset out"() -> (w501:i16)
        n198 = Scale By Power Of 2(n=7, x="shift integrator control") -> (x*2^n=w502:i32)
        n199 = Subtract(x=w501, y="offset retraction drift") -> (x-y=w500:i16)
        n200 = local write "shift integrator"(w502) -> ()
        n201 = local write "offset out"(w500) -> ()
      }
      frame #2 {
        n202 = call "Wait"("Count(uSec)"="time before averaging drift") -> ()  [unwired: 1 out]
      }
      frame #3 {
        n203 = for {
          N: "drift averager" -> [_]
          shift-right: [w516] -> w511
          shift-left: 0 -> [w517]
          n204 = local read "TF-drift"() -> (w514:i16)
          n205 = Add(x=w514, y=w517) -> (x+y=w516:i32)
          n206 = call "Loop Timer2"("Count(uSec)"="drift Waiting (uSec)") -> ()  [unwired: 1 out]
        }
        n207 = Quotient & Remainder(x=w511, y="drift averager") -> (floor(x/y)=w507:i32)  [unwired: 1 out]
        n208 = Subtract(x=w507, y="offset FM") -> (x-y=w508:i32)
        n209 = local write "Internal Setpoint Internal Control"(w508) -> ()
      }
      frame #4 {
        n210 = local write "Stop Feedback"(FALSE ("Stop Feedback")) -> ()
      }
      frame #5 {
        n211 = Set Occurrence(w520) -> ()
      }
    }
  }
  n212 = while {
    stop <- FALSE stop-if-true
    n213 = local read "X Output Value"() -> (w522:i16)
    n214 = local read "Y Output Value"() -> (w521:i16)
    n215 = xnode "FPGA I/O Node"("Connector0/AO3"=w521) -> ()  [unwired: 1 in, 1 out]
    n216 = xnode "FPGA I/O Node"("Connector0/AO0"=w522) -> ()  [unwired: 1 in, 1 out]
  }
  n217 = while {
    stop <- FALSE stop-if-true
    n218 = xnode "TF Out"() -> ("Connector0/AI5"=w525:i16)  [unwired: 1 in, 1 out]
    n219 = xnode "Butterworth Filter"("input data"=w525) -> ("output data"=→"AI5":fxp<+/-,20,20>)  [unwired: 2 in]
  }
  n220 = while {
    stop <- FALSE stop-if-true
    n221 = xnode "TF Out"() -> ("Connector0/AI2"=→"AI2":i16)  [unwired: 1 in, 1 out]
  }
  n222 = while {
    stop <- FALSE stop-if-true
    n223 = local read "Step"() -> (w539:bool)
    n224 = local read "En"() -> (w537:bool)
    n225 = local read "Dir"() -> (w538:bool)
    n226 = xnode "FPGA I/O Node"("Connector0/DIO3"=w537) -> ()  [unwired: 1 in, 1 out]
    n227 = xnode "FPGA I/O Node"("Connector0/DIO2"=w538) -> ()  [unwired: 1 in, 1 out]
    n228 = xnode "FPGA I/O Node"("Connector0/DIO4"=w539) -> ()  [unwired: 1 in, 1 out]
  }
  n229 = while {
    stop <- FALSE stop-if-true
    n230 = xnode "TF Out"() -> ("Connector0/AI7"=w541:i16)  [unwired: 1 in, 1 out]
    n231 = xnode "Butterworth Filter"("input data"=w541) -> ("output data"=→"TF-drift":fxp<+/-,20,20>)  [unwired: 2 in]
  }
  n232 = while {
    stop <- FALSE stop-if-true
    n233 = xnode "TF Out"() -> ("Connector0/AI6"=w551:i16)  [unwired: 1 in, 1 out]
    n234 = xnode "Butterworth Filter"("input data"=w551) -> ("output data"=→"AI6":fxp<+/-,20,20>)  [unwired: 2 in]
  }
  n235 = while {
    stop <- FALSE stop-if-true
    n236 = xnode "TF Out"() -> ("Connector0/AI4"=→"AI4":i16)  [unwired: 1 in, 1 out]
  }
